vi "Async.Engine.Start.vi"(8 "error in":errorcluster, 11 "Async in":refnum<class "VS Inline Async API (Express).lvclass">) -> (0 "error out":errorcluster, 3 "Async out":refnum<class "VS Inline Async API (Express).lvclass">)   [LabVIEW 2027, in "VS Inline Async API (Express).lvlib" / "VS Inline Async API (Express).lvclass"]
uses:
  VS Inline Async API (Express).lvclass
  VS Inline Async API (Express).lvclass/VS Inline Async API (Express).ctl
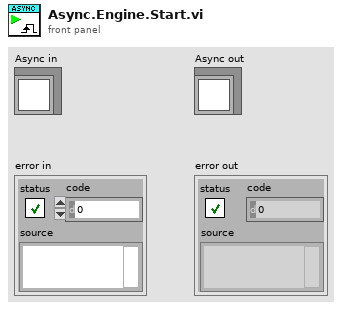
[diagram p1: front panel]
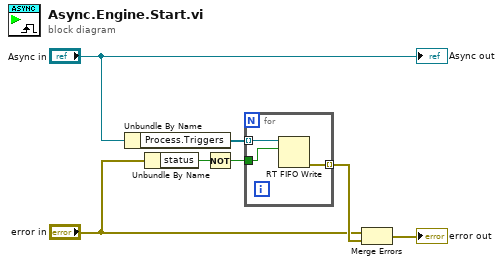
[diagram p0: block diagram]
diagram:
  n1 = Unbundle By Name("Async in") -> ("Process.Triggers"=w5:refnum<k33>[])
  n2 = Unbundle By Name("error in") -> ("status"=w3:bool)
  n3 = Not(x=w3) -> (.not. x?=w2:bool)
  n4 = for {
    tunnel: w5 -> [w10] mode=indexing
    tunnel: [w9] -> w7 mode=indexing
    tunnel: w2 -> [w8]
    n5 = RT FIFO Write(0:w10, 1:w8) -> (11:w9:errorcluster)  [unwired: 3 in, 3 out]
  }
  n6 = Merge Errors("error in", w7) -> (→"error out":errorcluster)
  "Async out" <- "Async in"
